vi "Error Message.vi"(0 "VISA resource name":refnum<visa-resource-name>, 5 "Type of Dialog (1: OK Msg)":i32(ring)=1 items=["No Dialog", "OK Message", "Continue or Stop Message"], 11 "error in (no error)":errorcluster) -> (3 "Status":bool, 4 "VISA resource name out":refnum<visa-resource-name>, 8 "Error Code (0)":i32, 10 "Error Message (empty)":string, 15 "error out":errorcluster)   [LabVIEW 2010, in "Yokogawa WT200 Series.lvlib"]
doc: "This VI contains all the intrument specific error codes and descriptions. Use this VI after executing several instrument driver VIs to recognize and display any errors that may have occurred."
uses:
  G:/Engineering/Retail/LabV/instr.lib/Yokogawa WT200 Series/Yokogawa WT200 Series.lvlib
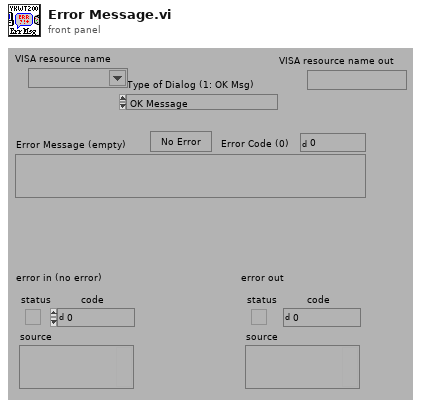
[diagram p1: front panel]
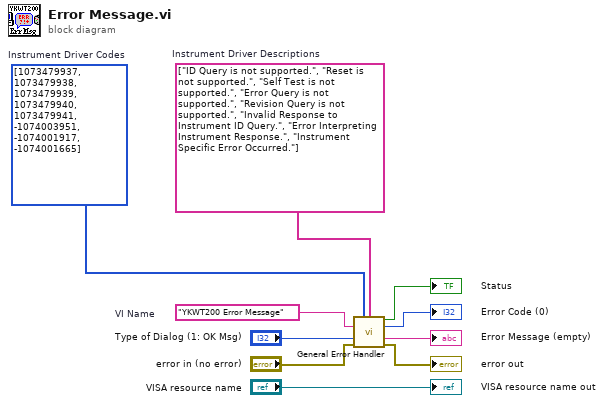
[diagram p0: block diagram]
diagram:
  w2 = i32[] [1073479937, 1073479938, 1073479939, 1073479940, 1073479941, -1074003951, -1074001917, -1074001665]  # Instrument Driver Codes
  w1 = string[] ["ID Query is not supported.", "Reset is not supported.", "Self Test is not supported.", "Error Query is not supported.", "Revision Query is not supported.", "Invalid Response to Instrument ID Query.", "Error Interpreting Instrument Response.", "Instrument Specific Error Occurred."]  # Instrument Driver Descriptions
  w7 = "YKWT200 Error Message"  # VI Name
  n1 = call <vilib>:"General Error Handler.vi"("[user-defined codes]"=w2, "[user-defined descriptions]"=w1, "[error source] (\" \")"=w7, "type of dialog (OK msg:1)"="Type of Dialog (1: OK Msg)", "error in (no error)"="error in (no error)") -> ("error?"=→"Status":bool, "code out"=→"Error Code (0)":i32, "message"=→"Error Message (empty)":string, "error out"=→"error out":errorcluster)  [unwired: 6 in, 1 out]
  "VISA resource name out" <- "VISA resource name"
